vi "Build Update Statement.vi"(8 "error in (no error)":errorcluster, 9 "TableType":T1, 10 "TableName Out":string, 11 "KDBConnection in":refnum<class "DBC.lvclass">) -> (0 "error out":errorcluster, 1 "Update Suffix Command":string, 2 "Table to Use":string, 3 "KDBConnection out":refnum<class "DBC.lvclass">)   [LabVIEW 2020, in "ORM_DBC_Kdb.lvlib" / "DBC.lvclass"]
uses:
  DBC.lvclass
  kdb_TableType_enum.ctl
  DBC.lvclass/DBC.ctl
  <vilib>/Utility/error.llb/Trim Whitespace.vi
  <vilib>/Utility/error.llb/Trim Whitespace One-Sided.vi
  <vilib>/Utility/file.llb/Is Path and Not Empty.vi
  <vilib>/Utility/error.llb/Error Cluster From Error Code.vi
  <vilib>/ErrorRing/Error Ring.xnode
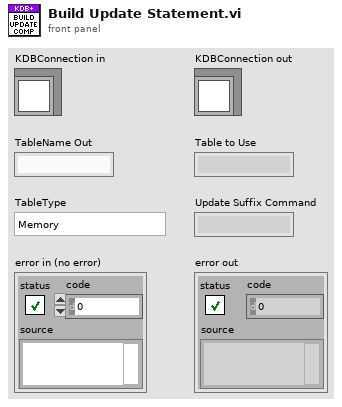
[diagram p1: front panel]
types:
  T1 = typedef "ORM_DBC_Kdb.lvlib/DBC.lvclass/kdb_TableType_enum.ctl" = enum16{"Memory", "Disk_Serialized", "Disk_Splayed", "Disk_Partitioned", "Other"}
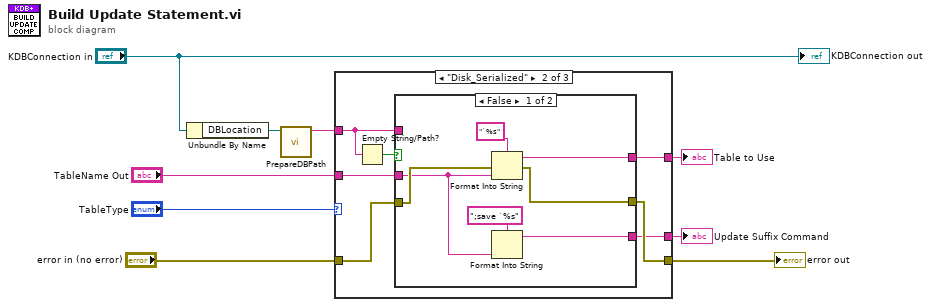
[diagram p0: block diagram]
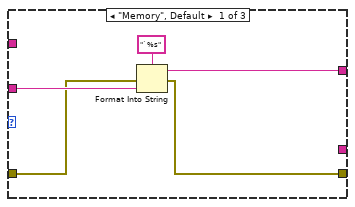
[diagram p2: hidden frame]
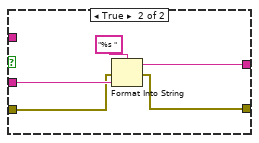
[diagram p3: hidden frame]
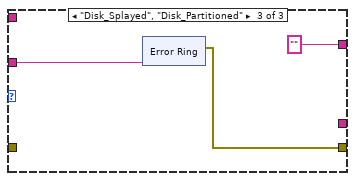
[diagram p4: hidden frame]
diagram:
  n1 = Unbundle By Name("KDBConnection in") -> ("DBLocation"=w9:path)
  n2 = call "PrepareDBPath.vi"("DBLocation"=w9) -> ("result string"=w8:string)  [unwired: 10 in]
  n3 = case shown="\"Disk_Serialized\"" "TableType" {
    tunnel: "TableName Out" -> [w14 w20 w36]
    tunnel: w8 -> [_ w19 _]
    tunnel: [w12 w21 ""] -> w2
    tunnel: "error in (no error)" -> [w11 w17 _]
    tunnel: [w10 w16 w34] -> w4
    tunnel: [_ w15 _] -> w1
    frame "Memory", Default {
      n4 = Format Into String(format string="`%s", error in=w11, w14) -> (resulting string=w12:string, error out=w10:errorcluster)  [unwired: 1 in]
    }
    frame "Disk_Serialized" {
      n5 = Empty String/Path?(string/path=w19) -> (empty?=w18:bool)
      n6 = case shown="False" w18 {
        tunnel: [w27 w31] -> w21
        tunnel: w20 -> [w22 w32]
        tunnel: w19 -> [_ _]
        tunnel: w17 -> [w26 w30]
        tunnel: [w25 w29] -> w16
        tunnel: [w23 _] -> w15
        frame False {
          n7 = Format Into String(format string="`%s", error in=w26, w22) -> (resulting string=w27:string, error out=w25:errorcluster)  [unwired: 1 in]
          n8 = Format Into String(format string=";save `%s", w22) -> (resulting string=w23:string)  [unwired: 2 in, 1 out]
        }
        frame True {
          n9 = Format Into String(format string="%s ", error in=w30, w32) -> (resulting string=w31:string, error out=w29:errorcluster)  [unwired: 1 in]
        }
      }
    }
    frame "Disk_Splayed", "Disk_Partitioned" {
      n10 = xnode "Error Ring"("parameter 0"=w36) -> ("error out"=w34:errorcluster)
    }
  }
  "error out" <- w4
  "Table to Use" <- w2
  "Update Suffix Command" <- w1
  "KDBConnection out" <- "KDBConnection in"
